vi "TestExec.Read Config for Executable and Args_V3.vi"(8 "error in":errorcluster, 10 "Vars":variant, 11 "Config File":path) -> (0 "error out":errorcluster, 1 "Args":string[](array[string]), 2 "Exe":path, 3 "Action Name":string, 4 "Error Code":i32, 6 "TimeOut":dbl)   [LabVIEW 2024]
uses:
  <vilib>/Utility/config.llb/Config Data RefNum.ctl
  Errors/Error.Error Code List.ctl
  <vilib>/Utility/config.llb/Read Key (Path).vi
  <vilib>/Utility/config.llb/Read Key (String).vi
  <vilib>/Utility/config.llb/Read Key (I32).vi
  <vilib>/Utility/config.llb/Read Key (Double).vi
  <vilib>/Utility/config.llb/NI_LVConfig.lvlib
  Errors.lvlib
  <vilib>/KATE/Files/File Utils.lvlib
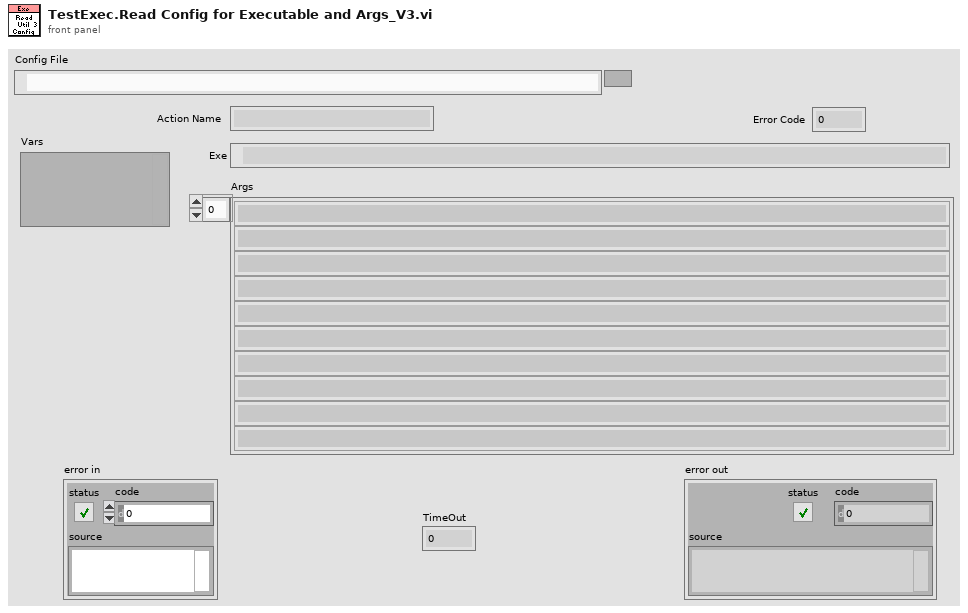
[diagram p1: front panel]
types:
  T1 = typedef "NI_LVConfig.lvlib/Config Data RefNum.ctl" = refnum<k1>
  T2 = cluster{"Exe":path, "Args":string[], "FileRef":T1, "Name":string, "Code":i32, "TimeOut":dbl}
  T3 = typedef "EQMF.lvlib/Errors.lvlib/Error.Error Code List.ctl" = i32
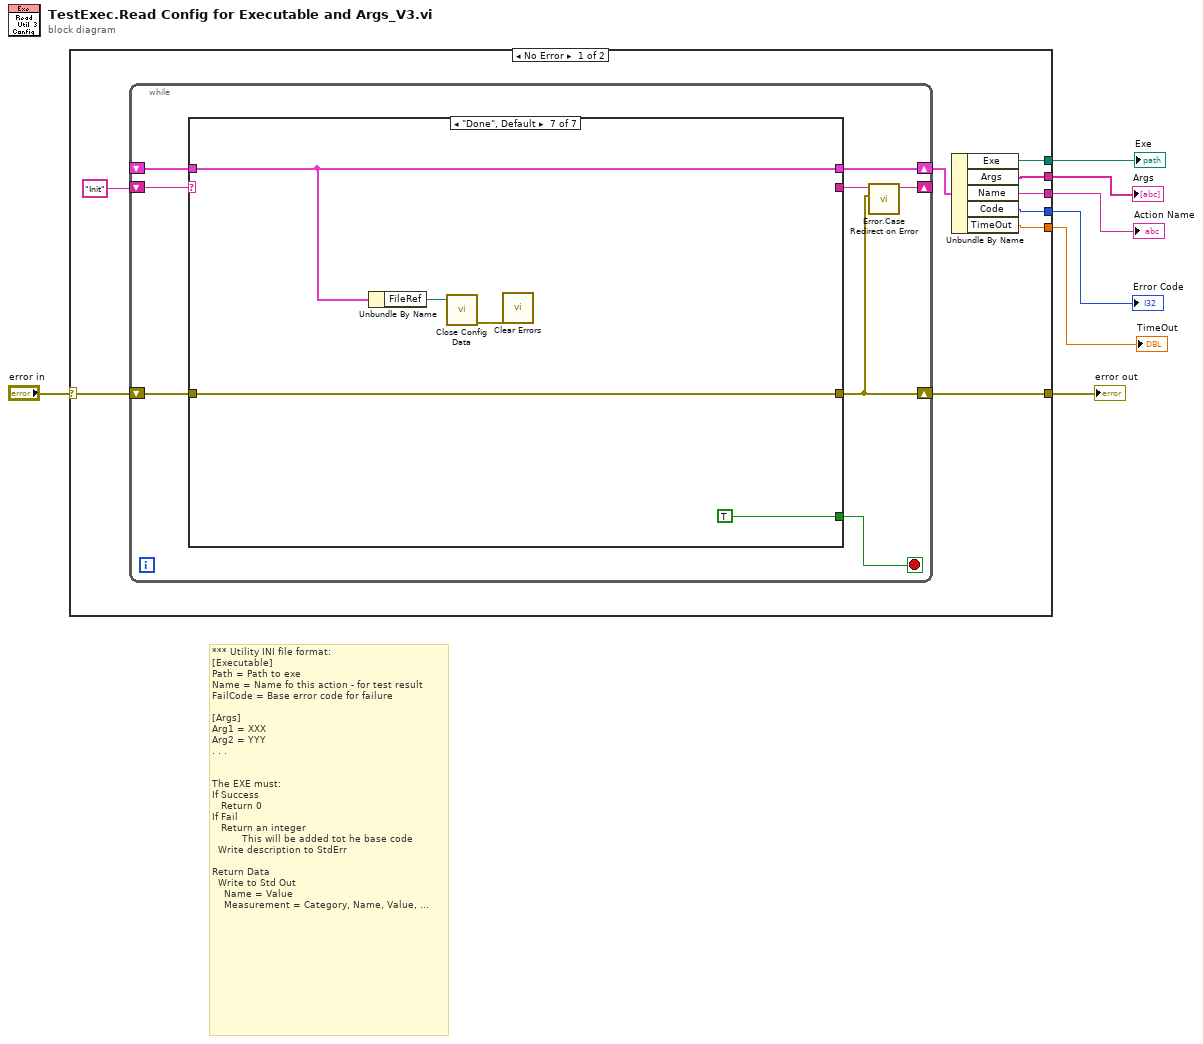
[diagram p0: block diagram]
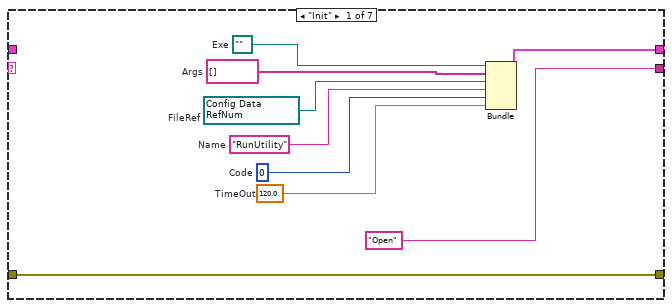
[diagram p2: hidden frame]
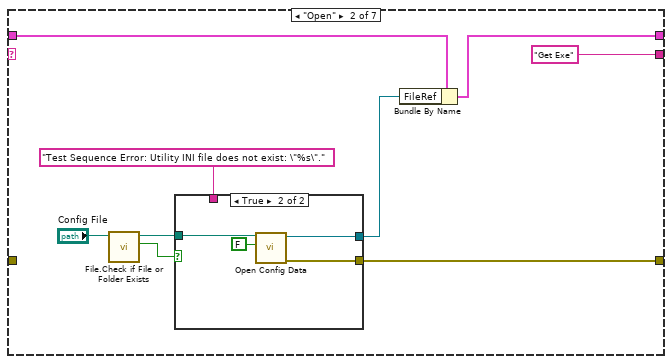
[diagram p3: hidden frame]
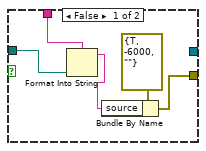
[diagram p4: hidden frame]
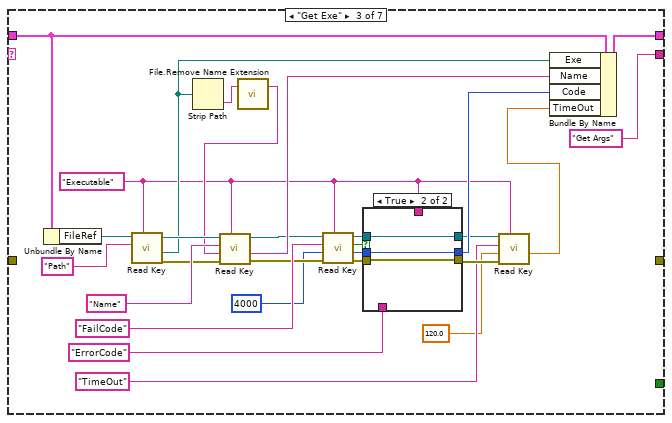
[diagram p5: hidden frame]
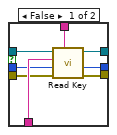
[diagram p6: hidden frame]
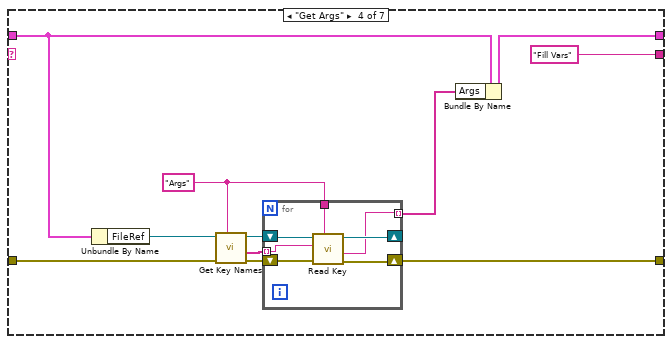
[diagram p7: hidden frame]
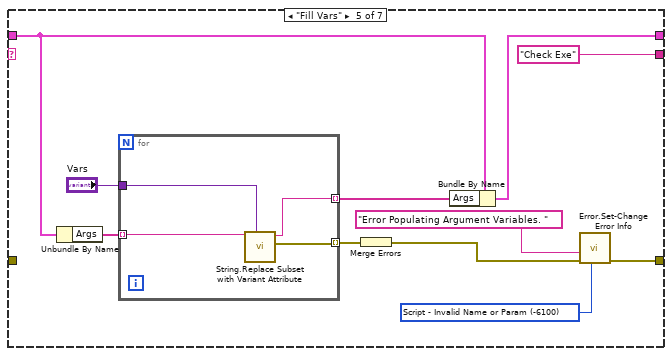
[diagram p8: hidden frame]
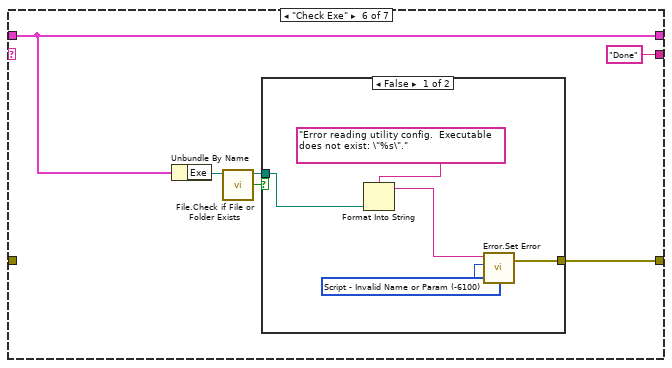
[diagram p9: hidden frame]
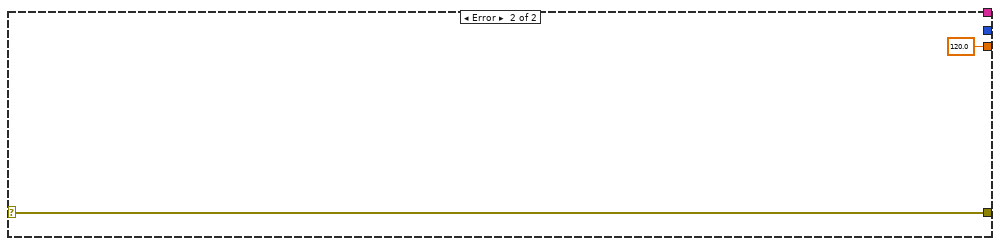
[diagram p11: hidden frame]
diagram:
  # "*** Utility INI file format:\n[Executable]\nPath = Path to exe\nName = Name fo this action - for test result\nFailCode = Base error code for failure \n\n[Args]\nArg1 = XXX\nArg2 = YYY\n. . . \n\n\nThe EXE must:\nIf Success\n   Return 0\nIf Fail\n   Return an integer\n          This will be added tot he base code\n  Write description to StdErr\n\nReturn Data\n  Write to Std Out\n    Name = Value\n    Measurement = Category, Name, Value, ..."
  n1 = case shown="No Error" "error in" {
    selector: "error in" -> [w15 w141]
    tunnel: [w12 _] -> w4
    tunnel: [w11 _] -> w7
    tunnel: [w14 w141] -> w6
    tunnel: [w10 _] -> w3
    tunnel: [w9 _] -> w2
    tunnel: [w8 120.0 ("TimeOut")] -> w1
    frame No Error {
      n2 = while {
        shift-right: [w22] -> w13
        shift-left: _ -> [w23]
        shift-right: [w21] -> _
        shift-left: "Init" -> [w24]
        shift-right: [w18] -> w14
        shift-left: w15 -> [w19]
        stop <- w17 stop-if-true
        n3 = case shown="\"Done\", Default" w24 {
          tunnel: w23 -> [_ w39 w78 w94 w114 w127 w138]
          tunnel: [w30 w40 w79 w95 w115 w127 w138] -> w22
          tunnel: ["Open" ("String") "Get Exe" ("String") "Get Args" ("String") "Fill Vars" ("String") "Check Exe" ("String") "Done" ("String") _] -> w20
          tunnel: w19 -> [w28 _ _ w97 _ _ w135]
          tunnel: [w28 w42 _ w96 w112 w128 w135] -> w18
          tunnel: [_ _ _ _ _ _ TRUE] -> w17
          frame "Init" {
            w25 = 120.0  # TimeOut
            w27 = "RunUtility"  # Name
            w26 = 0  # Code
            w31 = T1 refnum items=["config data"]  # FileRef
            w33 = path ""  # Exe
            w32 = string[] []  # Args
            n4 = Bundle("Exe"=w33, "Args"=w32, "FileRef"=w31, "Name"=w27, "Code"=w26, "TimeOut"=w25) -> (w30:T2)  [unwired: 1 in]
          }
          frame "Open" {
            n5 = call <vilib>:"File.Check if File or Folder Exists.vi"("Path"="Config File") -> ("Exists"=w35:bool, "Dup Path"=w36:path)  [unwired: 6 in, 3 out]
            n6 = case shown="True" w35 {
              tunnel: [w46 w51] -> w42
              tunnel: [_ w50] -> w41
              tunnel: w36 -> [w45 w49]
              tunnel: "Test Sequence Error: Utility INI file does not exist: \"%s\"." -> [w44 _]
              frame False {
                n7 = Format Into String(format string=w44, w45) -> (resulting string=w43:string)  [unwired: 2 in, 1 out]
                n8 = Bundle By Name(cluster=errorcluster {"status"=TRUE, "code"=-6000, "source"=""} ("error constant"), "source"=w43) -> (w46:errorcluster)
              }
              frame True {
                n9 = call <vilib>:"Open Config Data.vi"("create file if necessary (T)"=FALSE, "configuration file path"=w49) -> ("error out"=w51:errorcluster, "refnum"=w50:T1)  [unwired: 7 in, 1 out]
              }
            }
            n10 = Bundle By Name(cluster=w39, "FileRef"=w41) -> (w40:T2)
          }
          frame "Get Exe" {
            w54 = "Executable"
            n11 = Unbundle By Name(w78) -> ("FileRef"=w76:T1)
            n12 = call-poly <vilib>:"Read Key.vi"("section"=w54, "key"="Path", "refnum"=w76) -> ("error out"=w71:errorcluster, "value"=w69:path, "refnum out"=w74:T1)  [unwired: 5 in, 1 out]
            n13 = Strip Path(path=w69) -> (name=w68:string)  [unwired: 1 out]
            n14 = call <vilib>:"File.Remove Name Extension.vi"("File Name"=w68) -> ("Name Less Ext"=w67:string)  [unwired: 1 in, 1 out]
            n15 = call-poly <vilib>:"Read Key.vi"("section"=w54, "error in (no error)"=w71, "default value"=w67, "key"="Name", "refnum"=w74) -> ("error out"=w65:errorcluster, "value"=w70:string, "refnum out"=w66:T1)  [unwired: 3 in, 1 out]
            n16 = call-poly <vilib>:"Read Key.vi"("section"=w54, "error in (no error)"=w65, "default value"=4000, "key"="FailCode", "refnum"=w66) -> ("error out"=w60:errorcluster, "value"=w58:i32, "found?"=w61:bool, "refnum out"=w64:T1)  [unwired: 3 in]
            n17 = case shown="True" w61 {
              tunnel: w64 -> [w87 w89]
              tunnel: w54 -> [w86 _]
              tunnel: "ErrorCode" ("key") -> [w85 _]
              tunnel: w60 -> [w82 w88]
              tunnel: [w84 w90] -> w59
              tunnel: w58 -> [w83 w90]
              tunnel: [w81 w88] -> w56
              tunnel: [w80 w89] -> w57
              frame False {
                n18 = call-poly <vilib>:"Read Key.vi"("section"=w86, "error in (no error)"=w82, "default value"=w83, "key"=w85, "refnum"=w87) -> ("error out"=w81:errorcluster, "value"=w84:i32, "refnum out"=w80:T1)  [unwired: 3 in, 1 out]
              }
              frame True {
              }
            }
            n19 = call-poly <vilib>:"Read Key.vi"("section"=w54, "error in (no error)"=w56, "default value"=120.0, "key"="TimeOut", "refnum"=w57) -> ("value"=w53:dbl)  [unwired: 3 in, 3 out]
            n20 = Bundle By Name(cluster=w78, "Exe"=w69, "Name"=w70, "Code"=w59, "TimeOut"=w53) -> (w79:T2)
          }
          frame "Get Args" {
            w98 = "Args"
            n21 = Unbundle By Name(w94) -> ("FileRef"=w93:T1)
            n22 = call <vilib>:"Get Key Names.vi"("section"=w98, "error in (no error)"=w97, "refnum"=w93) -> ("error out"=w100:errorcluster, "key names"=w99:string[], "refnum out"=w101:T1)  [unwired: 5 in, 1 out]
            n23 = for {
              tunnel: w98 -> [w108]
              tunnel: w99 -> [w105] mode=indexing
              shift-right: [w104] -> _
              shift-left: w101 -> [w107]
              shift-right: [w103] -> w96
              shift-left: w100 -> [w106]
              tunnel: [w102] -> w92 mode=indexing
              n24 = call-poly <vilib>:"Read Key.vi"("section"=w108, "error in (no error)"=w106, "key"=w105, "refnum"=w107) -> ("error out"=w103:errorcluster, "value"=w102:string, "refnum out"=w104:T1)  [unwired: 4 in, 1 out]
            }
            n25 = Bundle By Name(cluster=w94, "Args"=w92) -> (w95:T2)
          }
          frame "Fill Vars" {
            w110 = T3 -6100 items=["No Error"=0, "Abort"=-2, "Misc"=-5000, "Fixture Error"=-5100, "File IO - General"=-5200, "FIle IO - Config Error"=-5201, "Instrument - General"=-5300, "Instrument - Serial Com"=-5301, "Instrument - Camera"=-5302, "Instrument - PS"=-5303, "Instrument - Oscilloscope"=-5304, "Instrument - Function Gen"=-5305, "Instrument - Load"=-5306, "Instrument - Meter"=-5307, "Instrument - Power Control"=-5308, "Instrument - Motion"=-5309, "Instrument - RF"=-5310, "System Exe"=-5400, "Image Processing"=-5500, "Communication"=-5600, "Script - Syntax Error"=-6000, "Script - Invalid Name or Param"=-6100, "Script - Timeout"=-6200, "Invalid Data"=-6300, "FW Update Error"=-6500] ("Std Code")
            n26 = Unbundle By Name(w114) -> ("Args"=w118:string[])
            n27 = for {
              tunnel: "Vars" -> [w123]
              tunnel: w118 -> [w122] mode=indexing
              tunnel: [w121] -> w117 mode=indexing
              tunnel: [w120] -> w116 mode=indexing
              n28 = call "String.Replace Subset with Variant Attribute.vi"("Vars"=w123, "Data In"=w122) -> ("error out"=w121:errorcluster, "Data Out"=w120:string)  [unwired: 8 in]
            }
            n29 = Merge Errors(w117) -> (w111:errorcluster)
            n30 = Bundle By Name(cluster=w114, "Args"=w116) -> (w115:T2)
            n31 = call "Error.Set-Change Error Info.vi"("Std Code"=w110, "error in"=w111, "Description"="Error Populating Argument Variables. ") -> ("error out"=w112:errorcluster)  [unwired: 8 in]
          }
          frame "Check Exe" {
            n32 = Unbundle By Name(w127) -> ("Exe"=w126:path)
            n33 = call <vilib>:"File.Check if File or Folder Exists.vi"("Path"=w126) -> ("Exists"=w125:bool, "Dup Path"=w124:path)  [unwired: 6 in, 3 out]
            n34 = case shown="False" w125 {
              tunnel: [w134 _] -> w128
              tunnel: w124 -> [w131 _]
              frame False {
                w133 = T3 -6100 items=["No Error"=0, "Abort"=-2, "Misc"=-5000, "Fixture Error"=-5100, "File IO - General"=-5200, "FIle IO - Config Error"=-5201, "Instrument - General"=-5300, "Instrument - Serial Com"=-5301, "Instrument - Camera"=-5302, "Instrument - PS"=-5303, "Instrument - Oscilloscope"=-5304, "Instrument - Function Gen"=-5305, "Instrument - Load"=-5306, "Instrument - Meter"=-5307, "Instrument - Power Control"=-5308, "Instrument - Motion"=-5309, "Instrument - RF"=-5310, "System Exe"=-5400, "Image Processing"=-5500, "Communication"=-5600, "Script - Syntax Error"=-6000, "Script - Invalid Name or Param"=-6100, "Script - Timeout"=-6200, "Invalid Data"=-6300, "FW Update Error"=-6500] ("Std Code")
                n35 = Format Into String(format string="Error reading utility config.  Executable does not exist: \"%s\"." ("Desc"), w131) -> (resulting string=w130:string)  [unwired: 2 in, 1 out]
                n36 = call "Error.Set Error.vi"("Std Code"=w133, "Desc"=w130) -> ("error out"=w134:errorcluster)  [unwired: 5 in]
              }
              frame True {
              }
            }
          }
          frame "Done", Default {
            n37 = Unbundle By Name(w138) -> ("FileRef"=w137:T1)
            n38 = call <vilib>:"Close Config Data.vi"("refnum"=w137) -> ("error out"=w136:errorcluster)  [unwired: 9 in, 1 out]
            n39 = call <vilib>:"Clear Errors.vi"("error in (no error)"=w136) -> ()  [unwired: 5 in, 2 out]
          }
        }
        n40 = call "Error.Case Redirect on Error.vi"("error in"=w18, "Next Case"=w20) -> ("Next Case Out"=w21:string)  [unwired: 9 in]
      }
      n41 = Unbundle By Name(w13) -> ("Exe"=w12:path, "Args"=w11:string[], "Name"=w10:string, "Code"=w9:i32, "TimeOut"=w8:dbl)
    }
    frame Error {
    }
  }
  "Exe" <- w4
  "Args" <- w7
  "error out" <- w6
  "Action Name" <- w3
  "Error Code" <- w2
  "TimeOut" <- w1
